vi "Enqueue Message.vi"(8 "error in (no error)":errorcluster, 10 "Queue Element In":refnum<class "TAS_Message.lvclass">, 11 "TAS_Message queue in":refnum<queue>) -> (0 "error out":errorcluster, 3 "TAS_Message queue out":refnum<queue>)   [LabVIEW 2012, in "TAS_Message.lvclass"]
uses:
  TAS_Message.lvclass
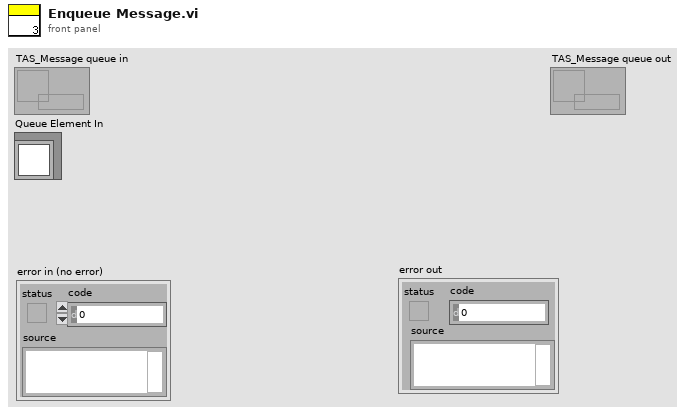
[diagram p1: front panel]
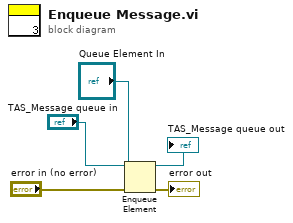
[diagram p0: block diagram]
diagram:
  n1 = Enqueue Element(queue="TAS_Message queue in", element="Queue Element In", error in (no error)="error in (no error)") -> (queue out=→"TAS_Message queue out":refnum<queue>, error out=→"error out":errorcluster)  [unwired: 1 in, 1 out]
